vi "Create RxTx.vi"(8 "error in (no error)":errorcluster, 11 "S4GEI in":refnum<class "S4GEI.lvclass">) -> (0 "error out":errorcluster, 3 "S4GEI out":refnum<class "S4GEI.lvclass">)   [LabVIEW 2018, in "S4GEI.lvclass"]
uses:
  S4GEI.lvclass
  S4GEI.lvclass/S4GEI.ctl
  RxTx/RxTx.lvclass
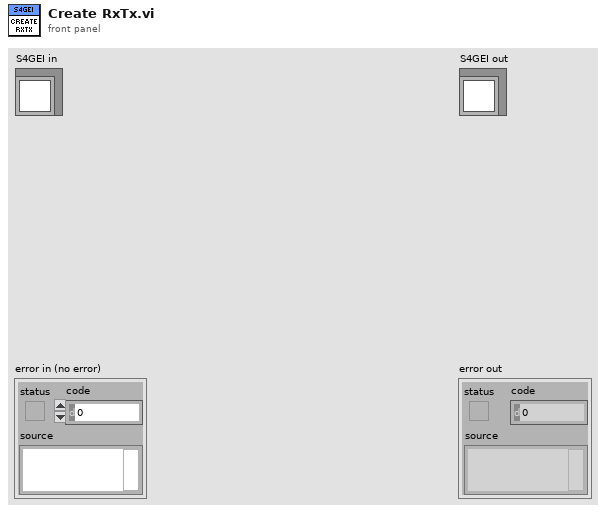
[diagram p1: front panel]
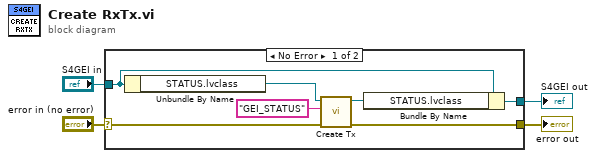
[diagram p0: block diagram]
diagram:
  n1 = case shown="No Error" "error in (no error)" {
    selector: "error in (no error)" -> [w10 w13]
    tunnel: [w9 w13] -> w3
    tunnel: [w7 w12] -> w1
    tunnel: "S4GEI in" -> [w8 w12]
    frame No Error {
      n2 = Unbundle By Name(w8) -> ("STATUS.lvclass"=w11:refnum<class "RxTx.lvclass">)
      n3 = call "Create Tx.vi"("error in (no error)"=w10, "Writer Name"="GEI_STATUS", "RxTx in"=w11) -> ("error out"=w9:errorcluster, "RxTx out"=w6:refnum<class "RxTx.lvclass">)  [unwired: 7 in]
      n4 = Bundle By Name(cluster=w8, "STATUS.lvclass"=w6) -> (w7:refnum<class "S4GEI.lvclass">)
    }
    frame Error {
    }
  }
  "error out" <- w3
  "S4GEI out" <- w1
